vi "Random Number Within Range.vi"   [LabVIEW 2009]
doc: "Generates a <b>Random Number</b> between <b>High</b> and <b>Low</b> inputs. Prechecks data to ensure that <b>High</b> is greater than <b>Low</b>."
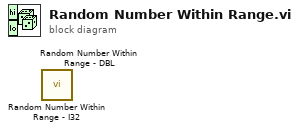
[diagram p0: block diagram]
diagram:
  n1 = call "Random Number Within Range - I32.vi"() -> ()  [unwired: 5 in, 1 out]
  n2 = call "Random Number Within Range - DBL.vi"() -> ()  [unwired: 5 in, 1 out]
